vi "Initialize Graph from logfile.vi"(8 "error in":errorcluster) -> (0 "error out":errorcluster, 2 "Data out":dbl[][](array[numeric]), 4 "Corrupt":bool)   [LabVIEW 2011]
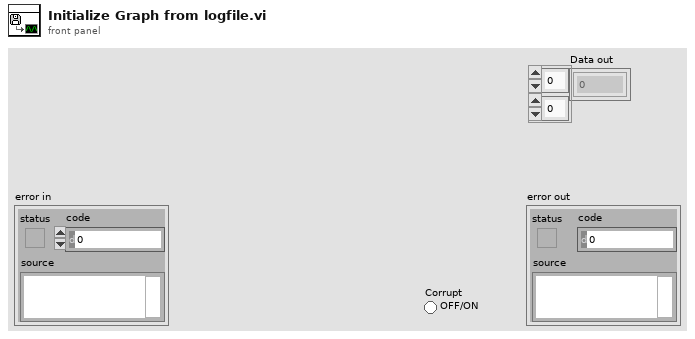
[diagram p1: front panel]
types:
  T1 = typedef "Log11 emibin file Metrix.ctl" = cluster{"data start":u32, "Bytes per package":i32, "Numb dbl":i32, "Numb u8 std":i32}
  T2 = typedef "User Setting Analog Channel Bg.ctl" = cluster{"Scaling":T3, "Limits and responces":T4, "Allow Graph selection by user":bool, "Unit":u16}
  T3 = typedef "Scaling.ctl" = cluster{"Gain":dbl, "Offset":dbl}
  T4 = typedef "Alarm Setup Analog.ctl" = cluster{"Technical Error(NA)":T5, "LL":T5, "L":T5, "H":T5, "HH":T5, "Limits":T7}
  T5 = typedef "Alarm Responce.ctl" = cluster{"Action":T6, "Alarm":bool}
  T6 = typedef "Action List.ctl" = enum16{"No Action", "Stop Motor", "Turn Off HV"}
  T7 = typedef "Limits.ctl" = cluster{"LL":dbl, "L":dbl, "H":dbl, "HH":dbl}
  T8 = typedef "Options  All pages and custom.ctl" = cluster{"P 1 (App)":T9, "P 2":T10, "P 3":T11, "P 4":T14, "P 5":T19, "P 6 (Err)":T20, "P 7 (Expert)":T21, "P 8 (Depth)":T23, "C 1":T24, "C 2":T25}
  T9 = typedef "Options Page 1 (App).ctl" = cluster{"Result files":path, "PCP Interface":string, "Tractor/Stroker Interface":string, "Tractor Interface":string, "Modem Status Interface":string, "Audible Alarm":bool, "Force alarm on Technical":bool, "Force alarm on HH":bool, "Force alarm on LL":bool, "Force alarm on H":bool, "Force alarm on L":bool}
  T10 = typedef "Options Page 2.ctl" = cluster{"Solenoid & Relay latching time":u16, "Tractor relay 1":dbl, "Tractor relay 2":dbl, "Tractor Solenoid limit":dbl}
  T11 = typedef "Options Page 3.ctl" = cluster{"Min resistance":dbl, "Max resistance":dbl, "Head voltage range":T12, "Max voltage jump":dbl, "Maximum resistance change":dbl, "Start Telemetry Voltage":dbl, "Start Telemetry Timeout":dbl, "Start Motor Voltage":dbl, "Stop Motor Voltage":dbl, "Pass Mode Warning Voltage":dbl, "Relay Switch Voltage":dbl, "Relay Status Loss Voltage":dbl, "Samples to average":i32, "PSU type DO NOT USE":T13, "Magna OVP":dbl, "Magna Current Limit":dbl}
  T12 = typedef "PCP type List.ctl" = enum16{"0 - 350V", "0 - 450V", "0 - 600V"}
  T13 = typedef "PSU Type.ctl" = enum16{"Unipower", "Magna 8.3A", "Magna 12A", "None"}
  T14 = typedef "Options Page 4.ctl" = cluster{"Solenoid & Relay latching time":u16, "Stroker relay 1":dbl, "Stroker Relay 2":dbl, "Stroker Solenoid limit":dbl, "Force det.":T15, "Stroke force lim.":dbl, "Anchor Enabled Pressure":dbl, "Tacometer puls":dbl, "Default anchor behavior":T16, "Default stroker behavior":T17, "Default stroker force limit (tonne)":dbl, "Slips Size":T18}
  T15 = typedef "Stroke force selector.ctl" = enum16{"Stroke in = node 1", "Strok out = node 1"}
  T16 = typedef "Default anchor behavior.ctl" = enum16{"Do nothing", "Set Anchor", "Release Anchor"}
  T17 = typedef "Default stroker behavior.ctl" = enum16{"Do nothing", "Stop", "Go Out", "Go In"}
  T18 = typedef "Slips Type Radio.ctl" = enum32{"No Selection", "338 MRS", "3,9 MRS"}
  T19 = typedef "Options Page 5.ctl" = cluster{"Solenoid & Relay latching time":u16, "Driller relay 1":dbl, "Driller Relay 2":dbl, "Driller  Solenoid limit":dbl}
  T20 = typedef "Options Page 6 (Err).ctl" = cluster{"Error and event files":path}
  T21 = typedef "Options Page 7 (Expert).ctl" = cluster{"Show Debug":bool, "Log debug messages":bool, "Additional debug messages":bool, "Start Beagle with Simulator data":bool, "Workshop mode":bool, "Modem baud":u16, "enumCANCOM":bool, "Modem sim":T22, "Telemetry Timeout Disable":i32, "Buffer size":i32, "Upd regular data":bool, "Cable comp":cluster{"VMOD1 Voltage(V)":dbl, "VMOD2 Voltage(V)":dbl}}
  T22 = typedef "Modem simulation setup.ctl" = cluster{"Modem dealay sim":bool, "Sim baud Tx":u16, "Bit Error fraction Tx":dbl, "Sim baud Rx":u16, "Bit Error fraction Rx":dbl}
  T23 = typedef "Options Page 8 (Depth).ctl" = cluster{"Winch Spool Circumference":dbl, "Winch Pulses per Revolution":dbl, "Current Depth":dbl}
  T24 = typedef "Options Custom 1.ctl" = cluster{"Depth Updated":bool, "Depth Offset":dbl}
  T25 = typedef "Options Custom 2.ctl" = cluster{"Placeholder":bool}
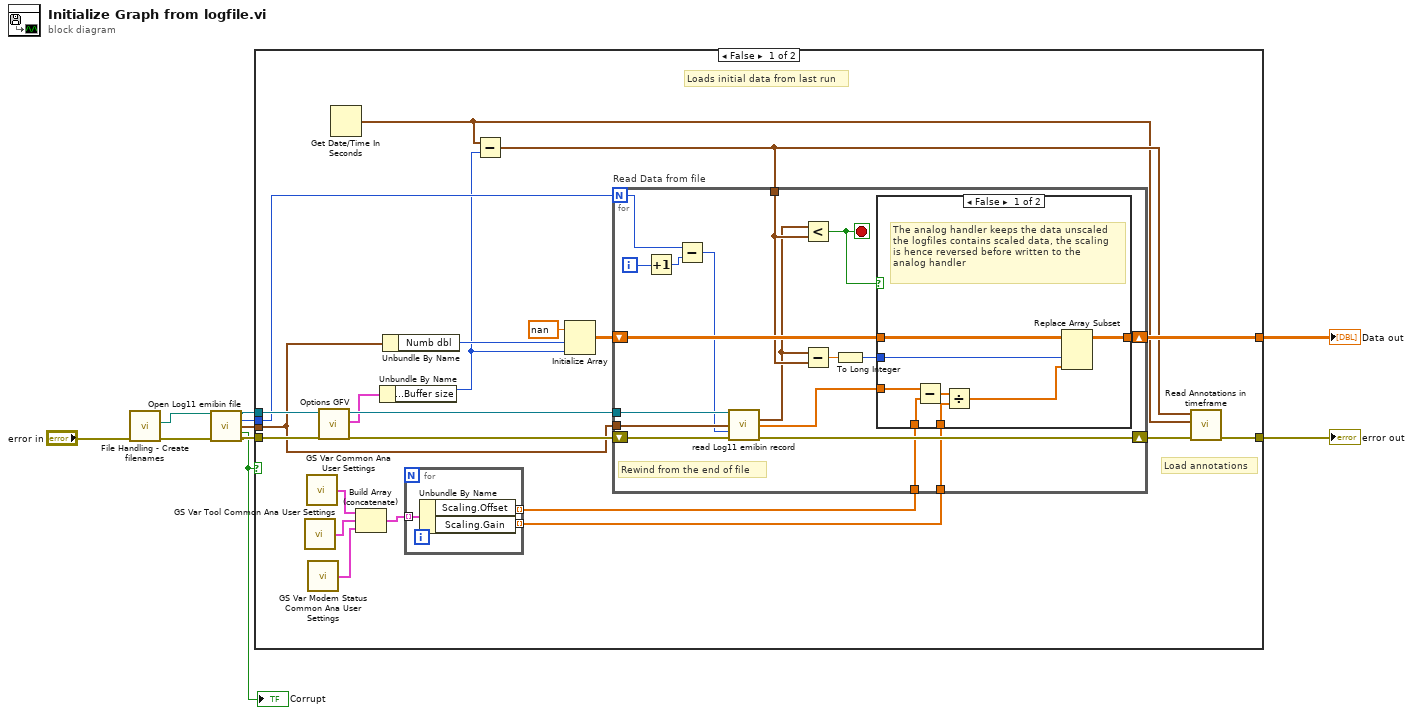
[diagram p0: block diagram]
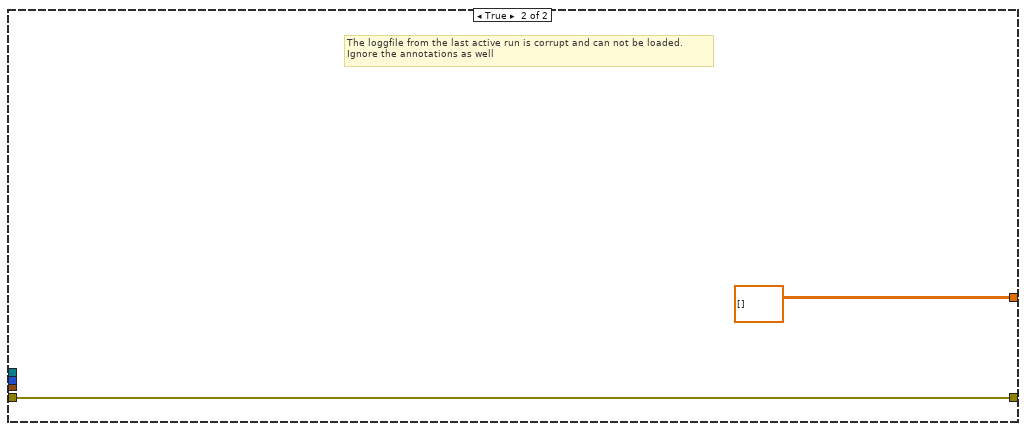
[diagram p3: hidden frame]
diagram:
  n1 = call "File Handling - Create filenames.vi"("error in"="error in") -> ("error out"=w6:errorcluster, "Binary Logfile path"=w7:path)  [unwired: 7 in, 2 out]
  n2 = call "Open Log11 emibin file.vi"("file path"=w7, "error in"=w6) -> ("refnum out"=w4:refnum<file>, "Numb packages"=w2:i64, "Log11 File Metrix"=w3:T1, "Corrupt"=w1:bool, "error out"=w5:errorcluster)  [unwired: 7 in, 2 out]
  "Corrupt" <- w1
  n3 = case shown="False" w1 {
    tunnel: w5 -> [w20 w62]
    tunnel: w4 -> [w28 _]
    tunnel: w3 -> [w17 _]
    tunnel: w2 -> [w27 _]
    tunnel: [w24 w62] -> w10
    tunnel: [w25 dbl[][] []] -> w9
    frame False {
      # "Load annotations"
      # "Loads initial data from last run"
      n4 = call "GS Var Tool Common Ana User Settings.vi"() -> ("Tool Analog var User settigns out"=w16:T2[])  [unwired: 13 in, 2 out]
      n5 = call "GS Var Common Ana User Settings.vi"() -> ("Common Analog var User set out"=w15:T2[])  [unwired: 13 in, 2 out]
      n6 = call "GS Var Modem Status Common Ana User Settings.vi"() -> ("Modem Status Analog var User settigns out"=w11:T2[])  [unwired: 13 in, 2 out]
      n7 = call "Options GFV.vi"("error in (no error)"=w20) -> ("Options"=w21:T8, "error out"=w18:errorcluster)  [unwired: 16 in, 1 out]
      n8 = Get Date/Time In Seconds() -> (seconds since 1Jan1904=w22:timestamp)
      n9 = Build Array (concatenate)(w15, w16, w11) -> (w14:T2[])
      n10 = Unbundle By Name(w21) -> ("P 7 (Expert).Buffer size"=w19:i32)
      n11 = Unbundle By Name(w17) -> ("Numb dbl"=w31:i32)
      n12 = for {
        tunnel: w14 -> [w34] mode=indexing
        tunnel: [w33] -> w13 mode=indexing
        tunnel: [w32] -> w12 mode=indexing
        n13 = Unbundle By Name(w34) -> ("Scaling.Offset"=w33:dbl, "Scaling.Gain"=w32:dbl)
      }
      n14 = Subtract(x=w22, y=w19) -> (x-y=w23:timestamp)
      n15 = Initialize Array(nan ("element"), w31, w19) -> (w30:dbl[][])
      n16 = for "Read Data from file" {
        N: w27 -> [w37]
        tunnel: w28 -> [w42]
        tunnel: w17 -> [w39]
        tunnel: w23 -> [w47]
        shift-right: [w49] -> w25
        shift-left: w30 -> [w48]
        shift-right: [w44] -> w26
        shift-left: w18 -> [w43]
        tunnel: w13 -> [w36]
        tunnel: w12 -> [w35]
        i -> [w52]
        stop <- w50 stop-if-true
        # "Rewind from the end of file"
        n17 = Increment(x=w52) -> (x+1=w51:i32)
        n18 = Subtract(x=w37, y=w51) -> (x-y=w38:i32)
        n19 = call "read Log11 emibin record.vi"("refnum in"=w42, "Log11 File Metrix"=w39, "Package(-1, Next)"=w38, "error in"=w43) -> ("record time"=w40:timestamp, "Doubles"=w41:dbl[], "error out"=w44:errorcluster)  [unwired: 7 in, 2 out]
        n20 = Less?(x=w40, y=w47) -> (x < y?=w50:bool)
        n21 = Subtract(x=w40, y=w47) -> (x-y=w46:dbl)
        n22 = To Long Integer(number=w46) -> (32bit integer=w45:i32)
        n23 = case shown="False" w50 {
          tunnel: [w59 w61] -> w49
          tunnel: w48 -> [w60 w61]
          tunnel: w41 -> [w57 _]
          tunnel: w45 -> [w58 _]
          tunnel: w36 -> [w55 _]
          tunnel: w35 -> [w54 _]
          frame False {
            # "The analog handler keeps the data unscaled\nthe logfiles contains scaled data, the scaling\nis hence reversed before written to the \nanalog handler"
            n24 = Subtract(x=w57, y=w55) -> (x-y=w56:dbl[])
            n25 = Divide(x=w56, y=w54) -> (x/y=w53:dbl[])
            n26 = Replace Array Subset(array=w60, new element=w53, index (col)=w58) -> (w59:dbl[][])  [unwired: 1 in]
          }
          frame True {
          }
        }
      }
      n27 = call "Read Annotations in timeframe.vi"("error in (no error)"=w26, "End Time"=w22, "Start Time"=w23) -> ("error out"=w24:errorcluster)  [unwired: 8 in]
    }
    frame True {
      # "The loggfile from the last active run is corrupt and can not be loaded.\nIgnore the annotations as well"
    }
  }
  "error out" <- w10
  "Data out" <- w9
